vi "TwoSensorMagazineLogic.vi"(0 "Intake Toggle":bool, 1 "Outtake Button":bool, 2 "Intake Side Sensor":bool, 3 "Outtake Side Sensor":bool, 4 "error in (no error)":errorcluster) -> (5 "Intake Motors":dbl, 6 "Magazine Motors":dbl, 7 "Kicker Motors":dbl, 8 "Intake Pistons":bool, 9 "error out":errorcluster)   [LabVIEW 2020]
uses:
  MagazineTest/MagazineControl.ctl
  TitanLib/Lib/TitanLib.lvlib
panel:
  out "Current State":T1
  in  "Kicker Power":dbl=0.5
  in  "Magazine Power":dbl=1.0
  in  "Input Power":dbl=1.0
  in  "Initial State":T1
  # "Inputs"
  # "Power Levels"
  # "Outputs"
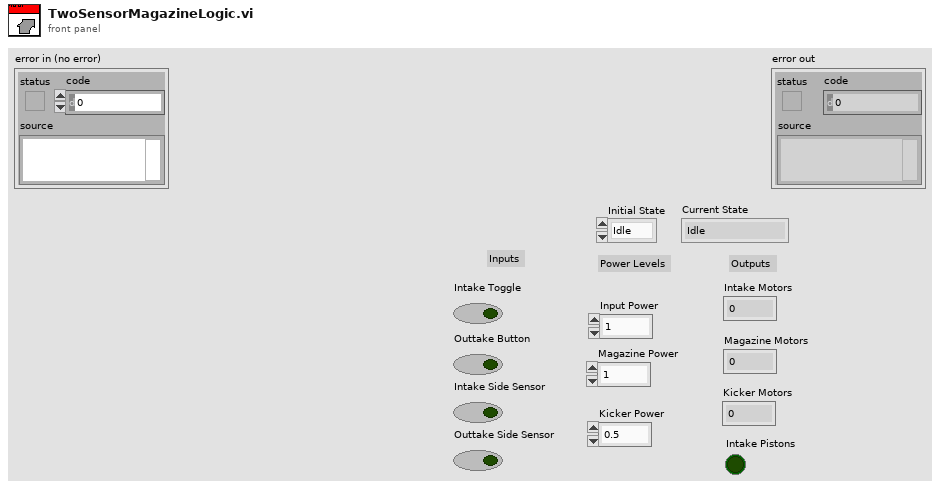
[diagram p1: front panel]
types:
  T1 = typedef "MagazineControl.ctl" = enum16{"Idle", "Intaking", "Outtake", "One Ball", "One Ball Intake", "One Ball Outtake", "Two Balls", "Two Ball Outtake"}
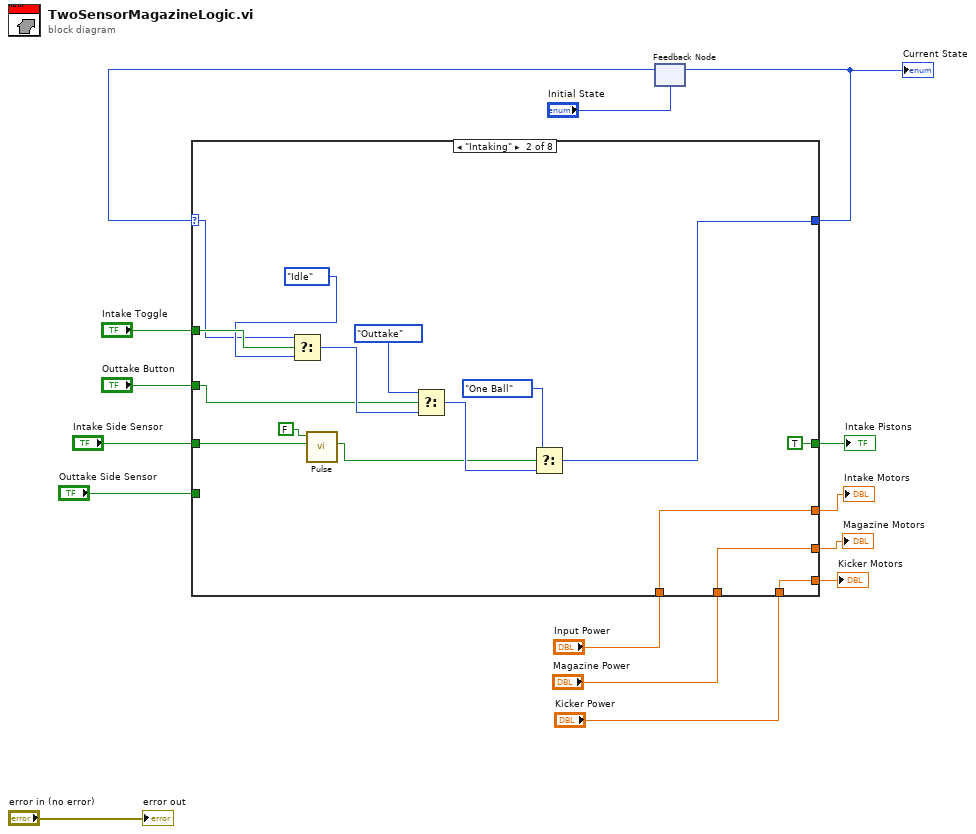
[diagram p0: block diagram]
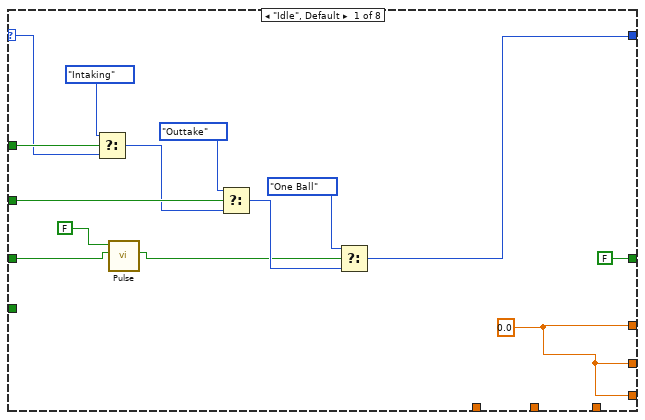
[diagram p2: hidden frame]
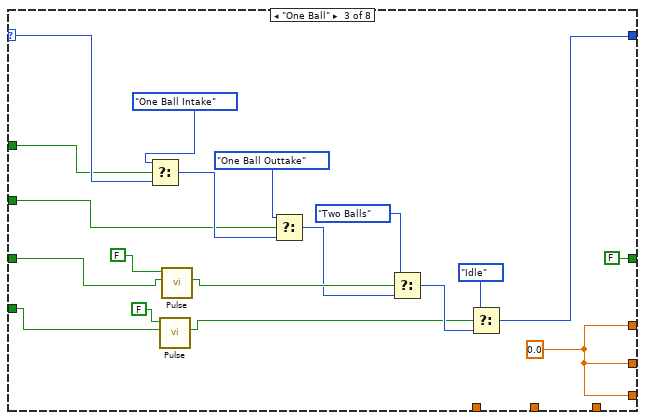
[diagram p3: hidden frame]
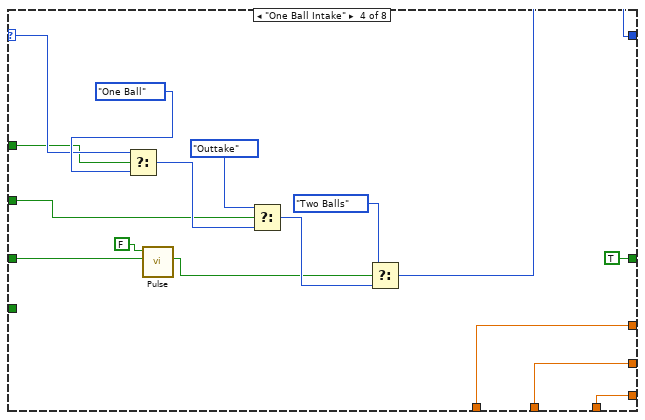
[diagram p4: hidden frame]
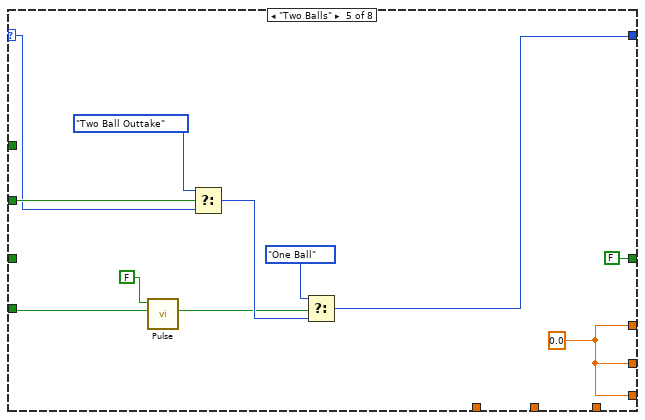
[diagram p5: hidden frame]
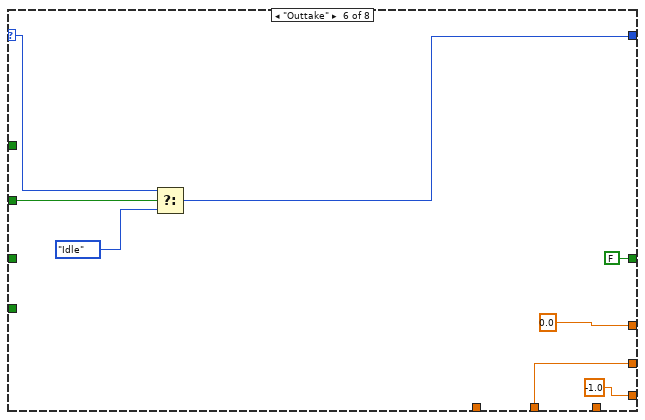
[diagram p6: hidden frame]
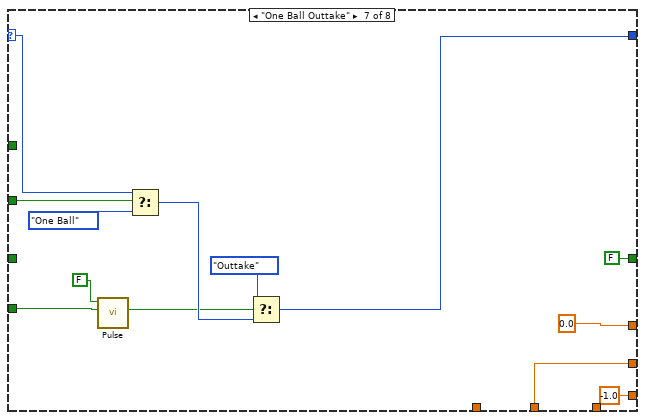
[diagram p7: hidden frame]
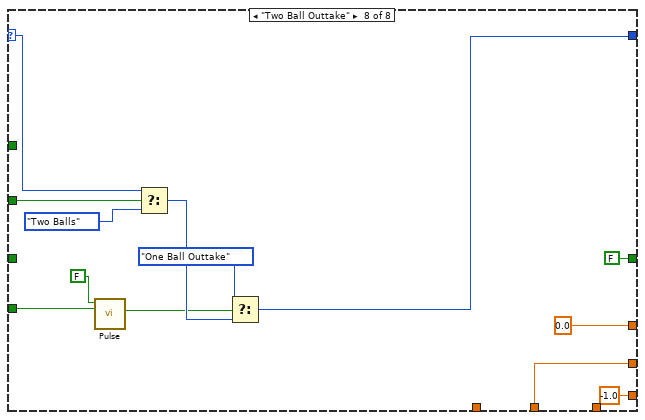
[diagram p8: hidden frame]
diagram:
  n1 = feedback #1("Initial State") -> (w4:T1)
  n2 = case shown="\"Intaking\"" w4 {
    selector: w4 -> [w25 w37 w55 w70 w90 w98 w108 w121]
    tunnel: "Intake Toggle" -> [w29 w40 w54 w69 _ _ _ _]
    tunnel: "Outtake Button" -> [w28 w39 w56 w71 w91 w99 w109 w122]
    tunnel: "Intake Side Sensor" -> [w19 w33 w57 w72 _ _ _ _]
    tunnel: [w21 w41 w50 w73 w87 w96 w104 w117] -> w3
    tunnel: [w17 w36 w53 w68 w88 0.0 ("Input Power") 0.0 ("Input Power") 0.0 ("Input Power")] -> w10
    tunnel: "Input Power" -> [_ w36 _ w68 _ _ _ _]
    tunnel: [w17 w35 w53 w67 w88 w93 w112 w125] -> w12
    tunnel: "Magazine Power" -> [_ w35 _ w67 _ w93 w112 w125]
    tunnel: [w17 w31 w53 w66 w88 -1.0 ("Kicker Motors") -1.0 ("Kicker Motors") -1.0 ("Kicker Motors")] -> w14
    tunnel: "Kicker Power" -> [_ w31 _ w66 _ _ _ _]
    tunnel: "Outtake Side Sensor" -> [_ _ w48 _ w83 _ w102 w116]
    tunnel: [FALSE ("Intake Pistons") TRUE ("Intake Pistons") FALSE ("Intake Pistons") TRUE ("Intake Pistons") FALSE ("Intake Pistons") FALSE ("Intake Pistons") FALSE ("Intake Pistons") FALSE ("Intake Pistons")] -> w2
    frame "Idle", Default {
      w17 = 0.0 ("Input Power")
      n3 = Select(t=MagazineControl."Intaking", s=w29, f=w25) -> (s? t:f=w27:T1)
      n4 = call "Pulse.vi"("Input"=w19, "Rising Edge?"=FALSE) -> ("Output"=w20:bool)  [unwired: 9 in]
      n5 = Select(t=MagazineControl."Outtake", s=w28, f=w27) -> (s? t:f=w26:T1)
      n6 = Select(t=MagazineControl."One Ball", s=w20, f=w26) -> (s? t:f=w21:T1)
    }
    frame "Intaking" {
      n7 = Select(t=w37, s=w40, f=MagazineControl."Idle" ("t")) -> (s? t:f=w44:T1)
      n8 = call "Pulse.vi"("Input"=w33, "Rising Edge?"=FALSE) -> ("Output"=w34:bool)  [unwired: 9 in]
      n9 = Select(t=MagazineControl."Outtake", s=w39, f=w44) -> (s? t:f=w45:T1)
      n10 = Select(t=MagazineControl."One Ball", s=w34, f=w45) -> (s? t:f=w41:T1)
    }
    frame "One Ball" {
      w53 = 0.0 ("Input Power")
      n11 = Select(t=MagazineControl."One Ball Intake", s=w54, f=w55) -> (s? t:f=w62:T1)
      n12 = call "Pulse.vi"("Input"=w48, "Rising Edge?"=FALSE) -> ("Output"=w47:bool)  [unwired: 9 in]
      n13 = call "Pulse.vi"("Input"=w57, "Rising Edge?"=FALSE) -> ("Output"=w64:bool)  [unwired: 9 in]
      n14 = Select(t=MagazineControl."One Ball Outtake", s=w56, f=w62) -> (s? t:f=w63:T1)
      n15 = Select(t=MagazineControl."Two Balls", s=w64, f=w63) -> (s? t:f=w52:T1)
      n16 = Select(t=MagazineControl."Idle", s=w47, f=w52) -> (s? t:f=w50:T1)
    }
    frame "One Ball Intake" {
      n17 = Select(t=w70, s=w69, f=MagazineControl."One Ball" ("t")) -> (s? t:f=w79:T1)
      n18 = call "Pulse.vi"("Input"=w72, "Rising Edge?"=FALSE) -> ("Output"=w75:bool)  [unwired: 9 in]
      n19 = Select(t=MagazineControl."Outtake", s=w71, f=w79) -> (s? t:f=w80:T1)
      n20 = Select(t=MagazineControl."Two Balls", s=w75, f=w80) -> (s? t:f=w73:T1)
    }
    frame "Two Balls" {
      w88 = 0.0 ("Input Power")
      n21 = call "Pulse.vi"("Input"=w83, "Rising Edge?"=FALSE) -> ("Output"=w84:bool)  [unwired: 9 in]
      n22 = Select(t=MagazineControl."Two Ball Outtake", s=w91, f=w90) -> (s? t:f=w86:T1)
      n23 = Select(t=MagazineControl."One Ball", s=w84, f=w86) -> (s? t:f=w87:T1)
    }
    frame "Outtake" {
      n24 = Select(t=w98, s=w99, f=MagazineControl."Idle") -> (s? t:f=w96:T1)
    }
    frame "One Ball Outtake" {
      n25 = call "Pulse.vi"("Input"=w102, "Rising Edge?"=FALSE) -> ("Output"=w103:bool)  [unwired: 9 in]
      n26 = Select(t=w108, s=w109, f=MagazineControl."One Ball") -> (s? t:f=w106:T1)
      n27 = Select(t=MagazineControl."Outtake", s=w103, f=w106) -> (s? t:f=w104:T1)
    }
    frame "Two Ball Outtake" {
      n28 = call "Pulse.vi"("Input"=w116, "Rising Edge?"=FALSE) -> ("Output"=w115:bool)  [unwired: 9 in]
      n29 = Select(t=w121, s=w122, f=MagazineControl."Two Balls") -> (s? t:f=w119:T1)
      n30 = Select(t=MagazineControl."One Ball Outtake", s=w115, f=w119) -> (s? t:f=w117:T1)
    }
  }
  "Intake Motors" <- w10
  "Magazine Motors" <- w12
  "Kicker Motors" <- w14
  "Current State" <- w3
  "Intake Pistons" <- w2
  n31 = feedback-in #1(w3) -> ()
  "error out" <- "error in (no error)"
